vi "Click Cycle_Set RW Row State.vi"(6 "Prior Property Array":T1(array[cluster]), 7 "Action":T2, 8 "Error In":errorcluster, 9 "Row RW State":T3, 10 "Active Item:Tag":string, 11 "All Tree Refs":refnum<vi>[](array[refnum])) -> (0 "Error Out":errorcluster, 3 "All Tree Refs Out":refnum<vi>[](array[refnum]))   [LabVIEW 2023]
uses:
  controls/action enum.ctl
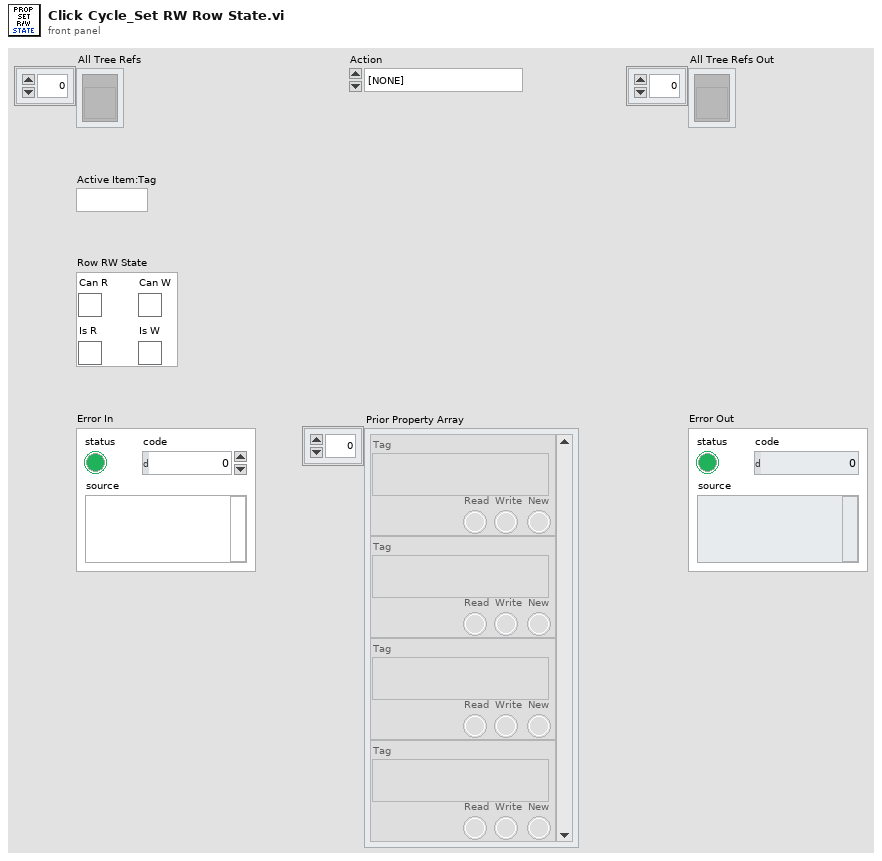
[diagram p1: front panel]
types:
  T1 = cluster{"Tag":string, "Read":bool, "Write":bool, "New":bool}[]
  T2 = typedef "action enum.ctl" = enum16{"[NONE]", "Wire Bundle", "Wire Unbundle", "Terminal Unbundle", "Terminal Bundle", "Bundler Move Up", "Bundler Move Down", "Bundler Insert", "Bundler Remove", "Bundler Remove Unwired", "Bundler Rearrange", "In Place Insert", "In Place Remove", "In Place Remove Unwired", "In Place Rearrange", "Wire Properties", "Wire Method", "Terminal Properties", "Terminal Method", "Property Move Up", "Property Move Down", "Properties Insert", "Properties Remove", "Properties Remove Unwired", "Properties Rearrange", "Method Change", "Class for Constant", "Class For Control", "Class For Node", "Class Name to Clipboard"}
  T3 = cluster{"Can R":bool, "Can W":bool, "Is R":bool, "Is W":bool}
  T4 = enum16{"[NONE]", "Wire Bundle", "Wire Unbundle", "Terminal Unbundle", "Terminal Bundle", "Bundler Insert", "Bundler Remove", "Bundler Remove Unwired", "Bundler Rearrange", "In Place Insert", "In Place Remove", "In Place Remove Unwired", "In Place Rearrange", "Wire Properties", "Wire Method", "Terminal Properties", "Terminal Method", "Properties Insert", "Properties Remove", "Properties Remove Unwired", "Properties Rearrange", "Method Change", "Class for Constant", "Class For Control", "Class For Node", "Class Name to Clipboard"}
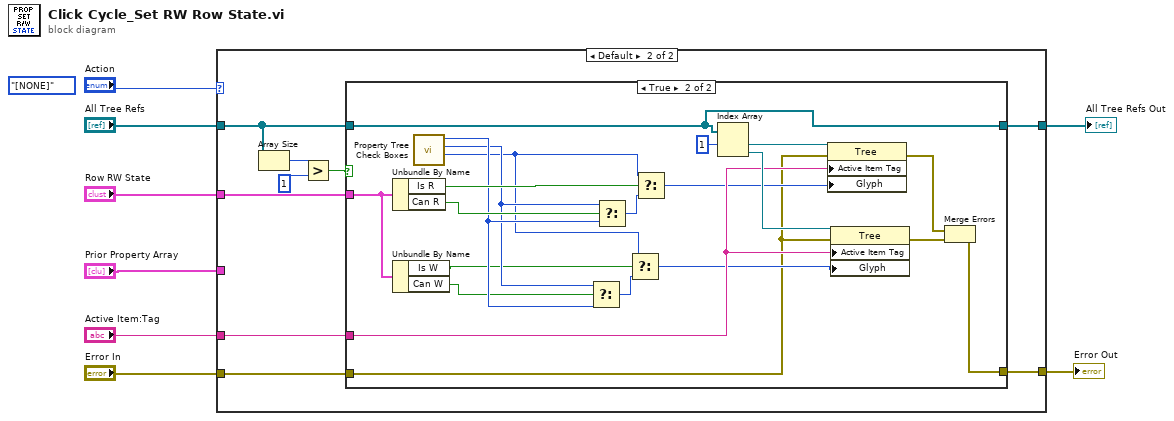
[diagram p0: block diagram]
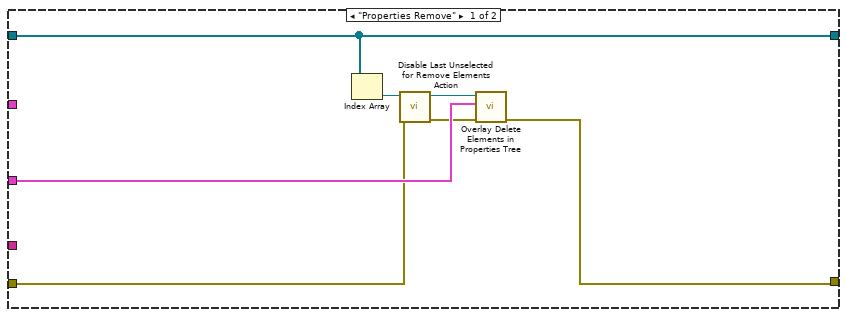
[diagram p2: hidden frame]
diagram:
  (unwired) T4."[NONE]" ("Action")
  n1 = case shown="Default" "Action" {
    tunnel: "Active Item:Tag" -> [_ w24]
    tunnel: "Row RW State" -> [_ w23]
    tunnel: [w13 w16] -> w6
    tunnel: "Error In" -> [w9 w22]
    tunnel: [w10 w21] -> w4
    tunnel: "All Tree Refs" -> [w13 w20]
    tunnel: "Prior Property Array" -> [w12 _]
    frame "Properties Remove" {
      n2 = Index Array(array=w13) -> (element=w14:refnum<vi>)  [unwired: 1 in]
      n3 = call "Disable Last Unselected for Remove Elements Action.vi"("error in"=w9, "Tree Ref"=w14) -> ("error out"=w11:errorcluster, "Tree Ref Out"=w15:refnum<vi>)  [unwired: 7 in, 1 out]
      n4 = call "Overlay Delete Elements in Properties Tree.vi"("error in"=w11, "Prior Property Array"=w12, "Tree Ref"=w15) -> ("error out"=w10:errorcluster)  [unwired: 7 in, 1 out]
    }
    frame Default {
      n5 = Array Size(array=w20) -> (size(s)=w19:i32)
      n6 = Greater?(x=w19, y=1) -> (0:w17:bool)
      n7 = case shown="True" w17 {
        tunnel: w24 -> [_ w44]
        tunnel: w23 -> [_ w32]
        tunnel: w22 -> [w25 w31]
        tunnel: [w25 w28] -> w21
        tunnel: w20 -> [w26 w27]
        tunnel: [w26 w27] -> w16
        frame False {
        }
        frame True {
          n8 = Unbundle By Name(w32) -> ("Is R"=w40:bool, "Can R"=w43:bool)
          n9 = Unbundle By Name(w32) -> ("Is W"=w34:bool, "Can W"=w33:bool)
          n10 = call "Property Tree Check Boxes.vi"() -> ("Checked"=w36:i32, "Unchecked"=w37:i32, "None"=w38:i32)  [unwired: 9 in]
          n11 = Select(t=w37, s=w33, f=w38) -> (s? t:f=w39:i32)
          n12 = Select(t=w37, s=w43, f=w38) -> (s? t:f=w42:i32)
          n13 = Select(t=w36, s=w34, f=w39) -> (s? t:f=w35:i32)
          n14 = Select(t=w36, s=w40, f=w42) -> (s? t:f=w41:i32)
          n15 = Index Array(array=w27, index #1=1 ("index")) -> (element #1=w46:refnum<vi>, element #2=w45:refnum<vi>)  [unwired: 1 in]
          n16 = property class="Tree"(reference=w46, error in=w31, "Active Item Tag"=w44, "Glyph"=w41) -> (error out=w29:errorcluster)  [unwired: 1 out]
          n17 = property class="Tree"(reference=w45, error in=w31, "Active Item Tag"=w44, "Glyph"=w35) -> (error out=w30:errorcluster)  [unwired: 1 out]
          n18 = Merge Errors(w29, w30) -> (w28:errorcluster)
        }
      }
    }
  }
  "All Tree Refs Out" <- w6
  "Error Out" <- w4
